vi "Actor Core.vi"(8 "error in":errorcluster, 11 "Aperiodic DAQ in":refnum<class "Aperiodic DAQ.lvclass">=refnum) -> (0 "error out":errorcluster, 3 "Actor out":refnum<class "Actor.lvclass">)   [LabVIEW 2014, in "Aperiodic DAQ.lvclass"]
doc: "(<B>Filename</B>: Actor Framework.lvlib:Actor.lvclass:Actor Core.vi)\n\nReceives messages to the actor, reacts to them, and initiates any error handling that may shut the actor down.\n\nDescendant classes may override this VI to append parallel tasks for the actor to complete while it handles messages. Overrides use the Call Parent Method node."
uses:
  Aperiodic DAQ.lvclass
  <vilib>/ActorFramework/Actor/Actor.lvclass
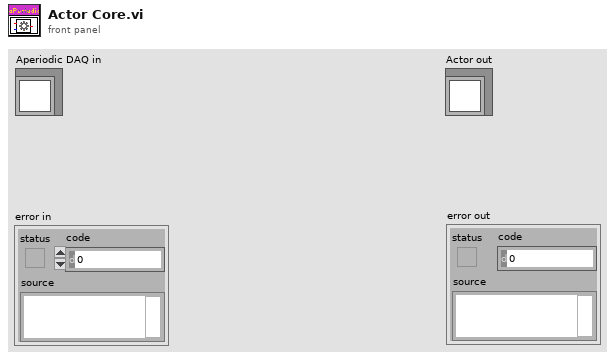
[diagram p1: front panel]
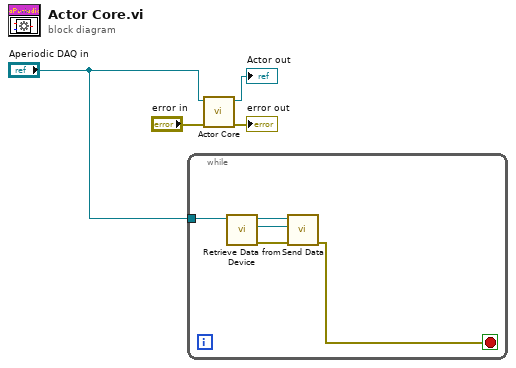
[diagram p0: block diagram]
diagram:
  n1 = while {
    tunnel: "Aperiodic DAQ in" -> [w9]
    stop <- w5 stop-if-true
    n2 = call-dynamic "Retrieve Data from Device.vi"("Aperiodic DAQ in"=w9) -> ("error out"=w7:errorcluster, "Data"=w6:refnum<class "Data.lvclass">, "Aperiodic DAQ out"=w8:refnum<class "Aperiodic DAQ.lvclass">)  [unwired: 8 in]
    n3 = call-dynamic "Send Data.vi"("error in"=w7, "Data"=w6, "DAQ Device in"=w8) -> ("error out"=w5:errorcluster)  [unwired: 7 in, 1 out]
  }
  n4 = call-parent "Actor Core.vi"("error in"="error in", "DAQ Device in"="Aperiodic DAQ in") -> ("error out"=→"error out":errorcluster, "Actor out"=→"Actor out":refnum<class "Actor.lvclass">)  [unwired: 8 in]
